vi "Collect Refs.vi"(8 "error in (no error)":errorcluster, 11 "Refs in":T1) -> (0 "error out":errorcluster, 3 "Refs":T1)   [LabVIEW 2020, in "FlexBlocks.lvlib"]
uses:
  FlexBlocks.lvlib
  Traverse for BD Refs.vi
  3c4a2764-9b1a-429d-a820-531ae47cea45.vi
  <vilib>/Utility/traverseref.llb/TRef TravTarget.ctl
  Scripting Refs.ctl
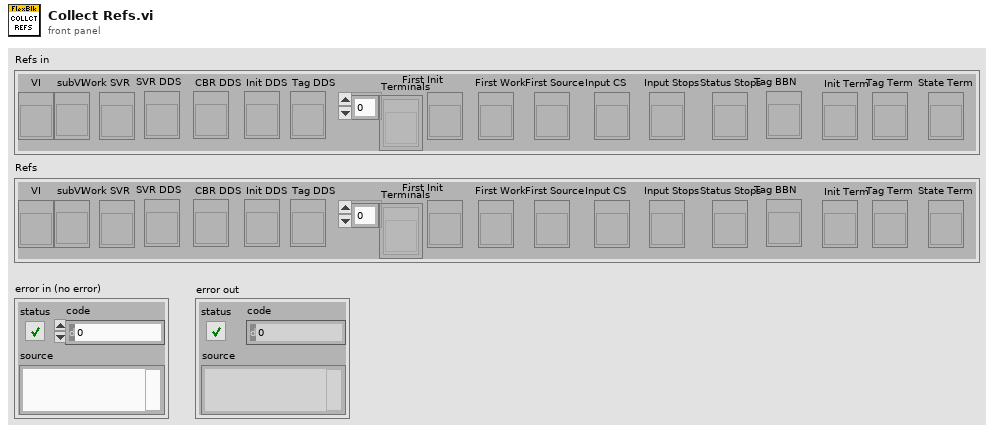
[diagram p1: front panel]
types:
  T1 = typedef "FlexBlocks.lvlib/Scripting Refs.ctl" = cluster{"VI":refnum<vi>, "subVI":refnum<vi>, "Work SVR":refnum<vi>, "SVR DDS":refnum<vi>, "CBR DDS":refnum<vi>, "Init DDS":refnum<vi>, "Tag DDS":refnum<vi>, "Terminals":refnum<vi>[], "First Init":refnum<vi>, "First Work":refnum<vi>, "First Source":refnum<vi>, "Input CS":refnum<vi>, "Input Stops":refnum<vi>, "Status Stops":refnum<vi>, "Tag BBN":refnum<vi>, "Init Term":refnum<vi>, "Tag Term":refnum<vi>, "State Term":refnum<vi>}
  T2 = typedef "TRef TravTarget.ctl" = enum16{"FP", "BD", "Other"}
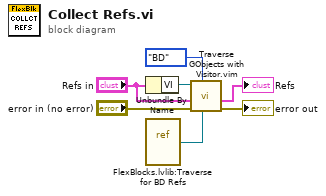
[diagram p0: block diagram]
diagram:
  n1 = Unbundle By Name("Refs in") -> ("VI"=w1:refnum<vi>)
  n2 = vi-ref "FlexBlocks.lvlib:Traverse for BD Refs.vi"() -> (w3:refnum<vi>)
  n3 = call "Traverse GObjects with Visitor.vim"("Visitor VI"=w3, "Traverse Target"=TRef_TravTarget."BD", "error in (no error)"="error in (no error)", "State in"="Refs in", "VI Ref in"=w1) -> ("error out"=→"error out":errorcluster, "State"=→"Refs":T1)  [unwired: 4 in, 1 out]
